vi "Calibrate Sonde Sensor.vi"(0 "RS232 Port In":refnum<visa-resource-name>="COM11", 1 "Calibration Standard":dbl, 3 "Calibrate command  string":string="XCP%+5.3f!", 5 "Sensor Address In":string="0", 9 "Calibrate":bool=TRUE, 11 "Error In (No Error)":errorcluster, 12 "Initialize/Close?":bool) -> (4 "RS232 Port Out":refnum<visa-resource-name>, 6 "Address Out":string, 8 "Calibration Response String":string, 10 "Sensor Calibrate Response":bool, 13 "Calibration Response":T1, 14 "Command":string, 15 "Error Out":errorcluster)   [LabVIEW 2016]
doc: "Sends an SDI-12 Send Identification Command, and returns the various attributes from the sensor's response.\n\nThe total size by the sensor must be 22-35 in size (inclusive), or this VI will return an error."
uses:
  SDI-12/SDI-12.lvlib
panel:
  out "read buffer":string
  # "(c) 2008 National Instruments.  ALL RIGHTS RESERVED."
  # "The following are required,\nor are optional, for the sensors\nto respond with:"
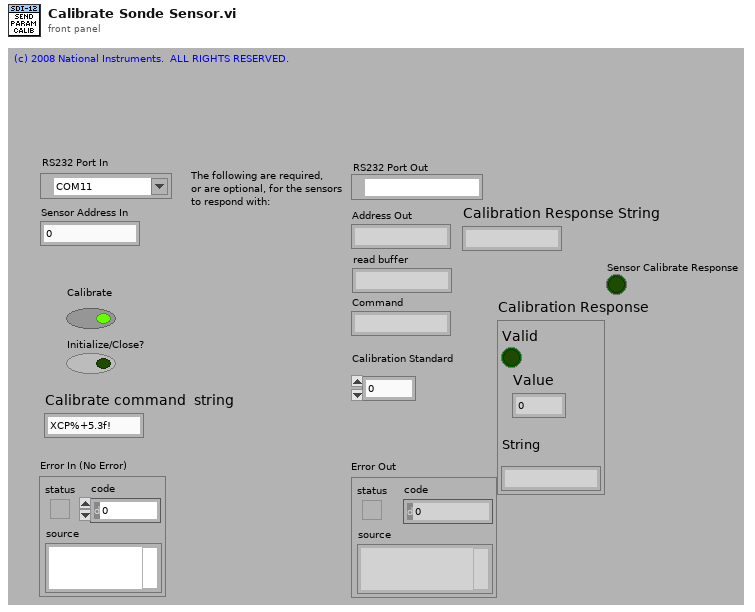
[diagram p1: front panel]
types:
  T1 = cluster{"Valid":bool, "Value":dbl, "\nString ":string}
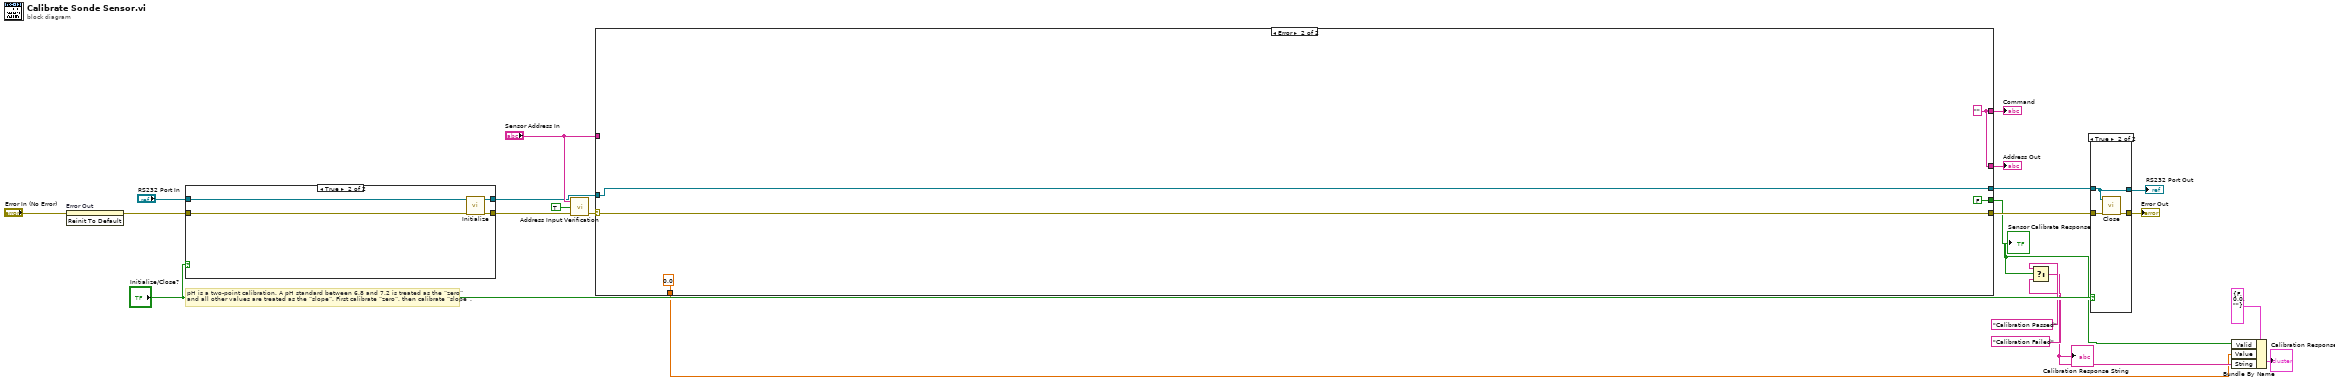
[diagram p0: block diagram]
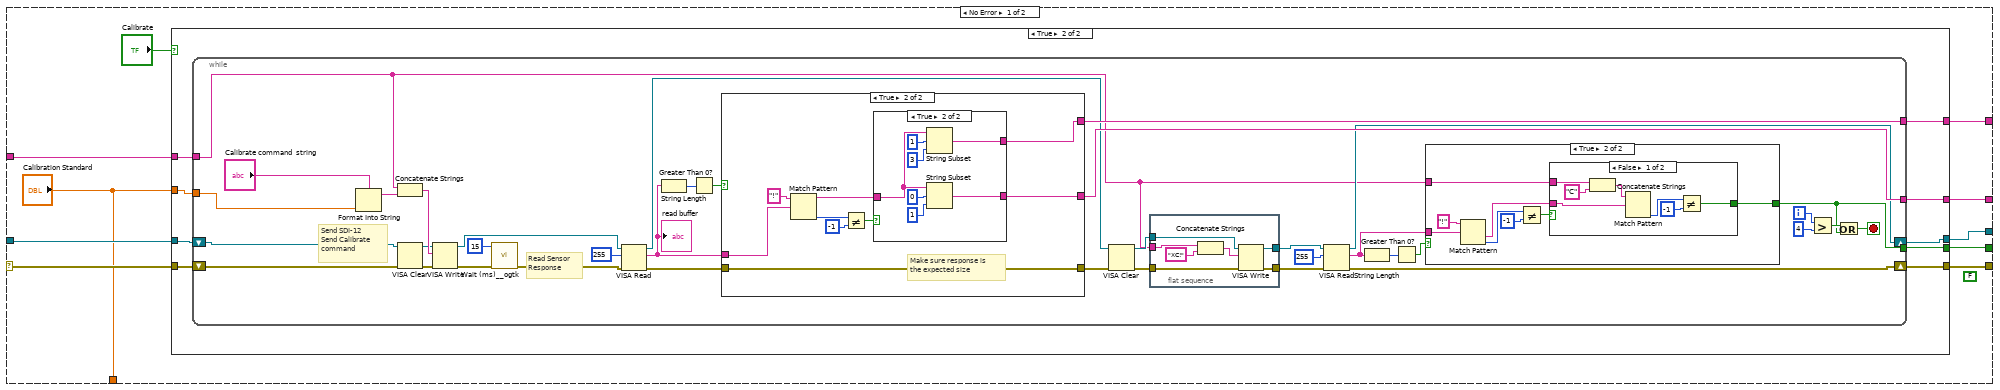
[diagram p4: hidden frame]
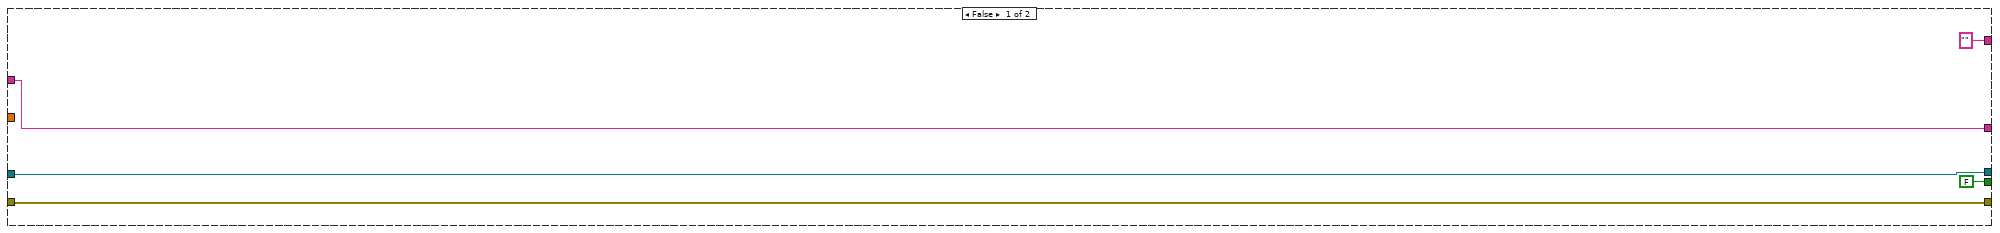
[diagram p5: hidden frame]
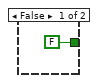
[diagram p6: hidden frame]
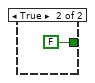
[diagram p7: hidden frame]
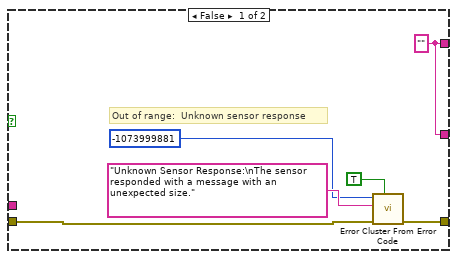
[diagram p8: hidden frame]
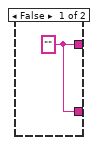
[diagram p9: hidden frame]
diagram:
  # "pH is a two-point calibration. A pH standard between 6.8 and 7.2 is treated as the “zero”\nand all other values are treated as the “slope”. First calibrate “zero”, then calibrate “slope”."
  n1 = invoke on="Error Out" class="Clust (strict)" method="Reinit To Default"(error in="Error In (No Error)") -> (error out=w8:errorcluster)  [unwired: 2 in, 2 out]
  n2 = case shown="True" "Initialize/Close?" {
    tunnel: w8 -> [w24 w28]
    tunnel: [w24 w27] -> w13
    tunnel: "RS232 Port In" -> [w23 w26]
    tunnel: [w23 w25] -> w11
    frame False {
    }
    frame True {
      n3 = call "Initialize.vi"("Error In (No Error)"=w28, "RS232 Port In"=w26) -> ("Error Out"=w27:errorcluster, "RS232 Port Out"=w25:refnum<visa-resource-name>)  [unwired: 8 in]
    }
  }
  n4 = call "Address Input Verification.vi"("Error In (No Error)"=w13, "Error if Bad? (True)"=TRUE ("error if bad? (True)"), "Sensor Address In (a)"="Sensor Address In") -> ("Error Out"=w22:errorcluster)  [unwired: 1 in, 1 out]
  n5 = case shown="Error" w22 {
    selector: w22 -> [w32 w141]
    tunnel: [w37 w141] -> w17
    tunnel: "Sensor Address In" -> [w31 _]
    tunnel: w11 -> [w30 w140]
    tunnel: [w38 w140] -> w14
    tunnel: [w36 w139] -> w18
    tunnel: [w35 w139] -> w19
    tunnel: [w34 FALSE] -> w3
    tunnel: ["Calibration Standard" 0.0 ("Calibration Standard")] -> w1
    frame No Error {
      (unwired) FALSE ("Initialize/Close?")
      n6 = case shown="True" "Calibrate" {
        tunnel: w31 -> [w41 w52]
        tunnel: w30 -> [w43 w51]
        tunnel: [w43 w50] -> w38
        tunnel: [w42 w49] -> w37
        tunnel: ["" ("read buffer") w48] -> w36
        tunnel: [w41 w47] -> w35
        tunnel: [FALSE w44] -> w34
        tunnel: w32 -> [w42 w46]
        tunnel: "Calibration Standard" -> [_ w45]
        frame False {
        }
        frame True {
          n7 = while {
            tunnel: w52 -> [w54]
            tunnel: [w83] -> w48
            tunnel: [w82] -> w47
            tunnel: w45 -> [w76]
            shift-right: [w59] -> w50
            shift-left: w51 -> [w85]
            shift-right: [w61] -> w49
            shift-left: w46 -> [w78]
            tunnel: [w53] -> w44
            i -> [w70]
            stop <- w58 stop-if-true
            # "Send SDI-12 \nSend Calibrate \ncommand"
            # "Read Sensor\nResponse"
            n8 = Format Into String(format string="Calibrate command  string", w76) -> (resulting string=w80:string)  [unwired: 2 in, 1 out]
            n9 = Concatenate Strings(w54, w80) -> (w86:string)
            n10 = VISA Clear(VISA resource name=w85, error in (no error)=w78) -> (VISA resource name out=w79:refnum<visa-resource-name>, error out=w77:errorcluster)
            n11 = VISA Write(VISA resource name=w79, write buffer=w86, error in (no error)=w77) -> (VISA resource name out=w89:refnum<visa-resource-name>, error out=w88:errorcluster)  [unwired: 1 out]
            n12 = call <userlib>:"Wait (ms)__ogtk.vi"("error in (no error)"=w88, "milliseconds to wait"=u32 15) -> ("error out"=w75:errorcluster)  [unwired: 8 in, 1 out]
            n13 = VISA Read(VISA resource name=w89, byte count=u32 255, error in (no error)=w75) -> (VISA resource name out=w66:refnum<visa-resource-name>, read buffer=w73:string, error out=w84:errorcluster)  [unwired: 1 out]
            "read buffer" <- w73
            n14 = String Length(string=w73) -> (length=w72:i32)
            n15 = Greater Than 0?(x=w72) -> (x > 0?=w71:bool)
            n16 = case shown="True" w71 {
              tunnel: w84 -> [w115 w128]
              tunnel: [w116 w128] -> w67
              tunnel: w73 -> [_ w120]
              tunnel: [w114 w127] -> w83
              tunnel: [w114 w126] -> w82
              frame False {
                w114 = "" ("read buffer")
                # "Out of range:  Unknown sensor response"
                n17 = call <vilib>:"Error Cluster From Error Code.vi"("show call chain? (False)"=TRUE, "error in (no error)"=w115, "error message (\"\")"="Unknown Sensor Response:\nThe sensor responded with a message with an unexpected size." ("error message (\"\")"), "error code (0)"=-1073999881) -> ("error out"=w116:errorcluster)  [unwired: 5 in]
              }
              frame True {
                # "Make sure response is\nthe expected size"
                n18 = Match Pattern(string="!", regular expression=w120) -> (before substring=w124:string, offset past match=w123:i32)  [unwired: 1 in, 2 out]
                n19 = Not Equal?(x=w123, y=-1) -> (x != y?=w122:bool)
                n20 = case shown="True" w122 {
                  tunnel: [w129 w133] -> w127
                  tunnel: [w129 w132] -> w126
                  tunnel: w124 -> [_ w131]
                  frame False {
                    w129 = "" ("string")
                  }
                  frame True {
                    n21 = String Subset(string=w131, offset (0)=1, length (rest)=3 ("length (rest)")) -> (substring=w133:string)
                    n22 = String Subset(string=w131, offset (0)=0, length (rest)=1 ("length (rest)")) -> (substring=w132:string)
                  }
                }
              }
            }
            n23 = VISA Clear(VISA resource name=w66, error in (no error)=w67) -> (VISA resource name out=w60:refnum<visa-resource-name>, error out=w62:errorcluster)
            n24 = flat-sequence {
              tunnel: [w96] -> w65
              tunnel: [w95] -> w64
              tunnel: w62 -> [w94]
              tunnel: w60 -> [w93]
              tunnel: w54 -> [w91]
              frame #0 {
                n25 = Concatenate Strings(w91, "XC!" ("string")) -> (w92:string)
                n26 = VISA Write(VISA resource name=w93, write buffer=w92, error in (no error)=w94) -> (VISA resource name out=w95:refnum<visa-resource-name>, error out=w96:errorcluster)  [unwired: 1 out]
              }
            }
            n27 = VISA Read(VISA resource name=w64, byte count=u32 255, error in (no error)=w65) -> (VISA resource name out=w59:refnum<visa-resource-name>, read buffer=w55:string, error out=w61:errorcluster)  [unwired: 1 out]
            n28 = String Length(string=w55) -> (length=w57:i32)
            n29 = Greater Than 0?(x=w57) -> (x > 0?=w56:bool)
            n30 = case shown="True" w56 {
              tunnel: w55 -> [_ w102]
              tunnel: w54 -> [_ w99]
              tunnel: [FALSE w98] -> w53
              frame False {
              }
              frame True {
                n31 = Match Pattern(string="!", regular expression=w102) -> (after substring=w100:string, offset past match=w104:i32)  [unwired: 1 in, 2 out]
                n32 = Not Equal?(x=w104, y=-1) -> (x != y?=w101:bool)
                n33 = case shown="False" w101 {
                  tunnel: w100 -> [w110 _]
                  tunnel: w99 -> [w107 _]
                  tunnel: [w106 FALSE] -> w98
                  frame False {
                    n34 = Concatenate Strings(w107, "C" ("string")) -> (w108:string)
                    n35 = Match Pattern(string=w108, regular expression=w110) -> (offset past match=w112:i32)  [unwired: 1 in, 3 out]
                    n36 = Not Equal?(x=w112, y=-1) -> (x != y?=w106:bool)
                  }
                  frame True {
                  }
                }
              }
            }
            n37 = Greater?(x=w70, y=4) -> (0:w68:bool)
            n38 = Or(x=w68, y=w53) -> (x .or. y?=w58:bool)
          }
        }
      }
    }
    frame Error {
      w139 = "" ("read buffer")
    }
  }
  "Command" <- w18
  "Address Out" <- w19
  "Sensor Calibrate Response" <- w3
  n39 = Select(t="Calibration Passed", s=w3, f="Calibration Failed") -> (s? t:f=w2:string)
  "Calibration Response String" <- w2
  n40 = case shown="True" "Initialize/Close?" {
    tunnel: w17 -> [w143 w146]
    tunnel: [w143 w145] -> w16
    tunnel: w14 -> [w142 w144]
    tunnel: [w142 w144] -> w15
    frame False {
    }
    frame True {
      n41 = call "Close.vi"("Error In (No Error)"=w146, "RS232 Port In"=w144) -> ("Error Out"=w145:errorcluster)  [unwired: 9 in]
    }
  }
  "Error Out" <- w16
  "RS232 Port Out" <- w15
  n42 = Bundle By Name(cluster=T1 {"Valid"=FALSE, "Value"=0.0, "\nString "=""} ("Calibration Response"), "Valid"=w3, "Value"=w1, "String"=w2) -> (→"Calibration Response":T1)
